vi "SUB-자료변환-실수형(float) 데이터를 32Bit 데이터로 변환.vi"(3 "FP32":sgl) -> (1 "INT32U":u32)   [LabVIEW 2015]
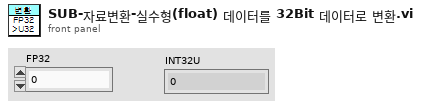
[diagram p1: front panel]
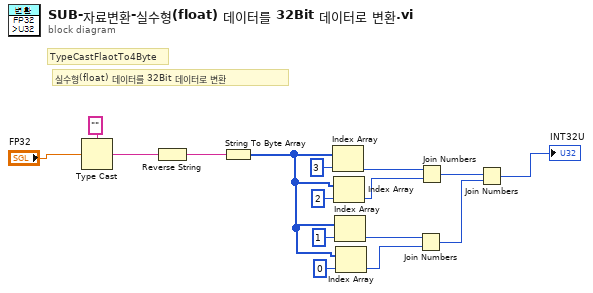
[diagram p0: block diagram]
diagram:
  # "실수형(float) 데이터를 32Bit 데이터로 변환"
  # "TypeCastFlaotTo4Byte"
  n1 = Type Cast(type="" ("타입"), x="FP32") -> (*(type *) &x=w16:string)
  n2 = Reverse String(1:w16) -> (0:w15:string)
  n3 = String To Byte Array(string=w15) -> (unsigned byte array=w10:u8[])
  n4 = Index Array(array=w10, index=3 ("인덱스")) -> (element=w9:u8)
  n5 = Index Array(array=w10, index=2 ("인덱스")) -> (element=w8:u8)
  n6 = Index Array(array=w10, index=1 ("인덱스")) -> (element=w7:u8)
  n7 = Index Array(array=w10, index=0 ("인덱스")) -> (element=w6:u8)
  n8 = Join Numbers(hi=w7, lo=w6) -> ((hi.lo)=w4:u16)
  n9 = Join Numbers(hi=w9, lo=w8) -> ((hi.lo)=w5:u16)
  n10 = Join Numbers(hi=w5, lo=w4) -> ((hi.lo)=→"INT32U":u32)
